vi "Geometry prep.vi"() -> ()   [LabVIEW 2015]
uses:
  <vilib>/Analysis/NI_AALPro.lvlib
panel:
  out "Area vectors, flap (sorted)":sgl[][](array[numeric])=[[-0.030221105, 0.0050799865, 0.0], [-0.025013696, 0.010133014, 0.0], [-0.016425999, 0.015131993, 0.0], [-0.004751401, 0.020000994, 0.0], [0.0092555005, 0.009600005, -0.0], [0.011616802, -0.009600005, 0.0], [0.017089, -0.020627992, 0.0], [0.038450897, -0.029717995, 0.0]]
  out "Area vectors, wing (sorted)":sgl[][](array[numeric])=[[-0.0203481, 0.080010995, 0.0], [-0.0011855003, 0.03999, 0.0], [0.0039664, 0.039116003, -0.0], [0.0067474004, 0.030846998, -0.0], [0.007422101, 0.019963002, -0.0], [0.005573, 0.009961, -0.0], [0.0017389987, 0.0023479997, -0.0], [0.0026417004, 0.0030260002, -0.0], [0.0037459005, 0.003527, -0.0], [0.0068250997, 0.002781997, -0.0], [0.0076412004, -0.0055579967, 0.0], [0.0006181995, -0.0030020003, 0.0], [-1.3899662e-05, -0.0030160001, 0.0], [-0.0003820001, -0.0030109999, 0.0], [-0.0011917998, -0.006011999, 0.0], [-0.0017578002, -0.0068530007, 0.0], [-0.0058059003, -0.022149, 0.0], [-0.0077515002, -0.039984, 0.0], [-0.0046135993, -0.039992005, 0.0], [-0.0017817, -0.03999, 0.0], [0.0030151003, -0.03999099, 0.0], [-0.0051033013, -0.022013, 0.0]]
  in  "Span (m)":dbl=1.0
  in  "Chord (m)":dbl=0.314309
  in  "Clockwise winding?":bool=TRUE
  in  "y/c flap (sorted)":dbl[](array[numeric])=[0.37029770016670227, 0.27414676547050476, 0.194563627243042, 0.1423029601573944, 0.12718598544597626, 0.15663312375545502, 0.19359293580055237, 0.24796299636363983]
  in  "x/c flap (sorted)":dbl[](array[numeric])=[0.9951130747795105, 0.9789506793022156, 0.9467116594314575, 0.8985679745674133, 0.8349331617355347, 0.8043899536132812, 0.8349331617355347, 0.9005628228187561]
  in  "y/c wing (sorted":dbl[](array[numeric])=[-0.055548522621393204, -0.12028767913579941, -0.12405944615602493, -0.1114400178194046, -0.0899726077914238, -0.06635858118534088, -0.04862762242555618, -0.043094854801893234, -0.034690067172050476, -0.022772176191210747, -0.0010575579944998026, 0.0232535507529974, 0.02522040344774723, 0.02517618052661419, 0.023960815742611885, 0.020169006660580635, 0.014576420187950134, -0.0038955300115048885, -0.028557566925883293, -0.04323611408472061, -0.04890473932027817, -0.03931194916367531]
  in  "x/c wing (sorted)":dbl[](array[numeric])=[0.7367812991142273, 0.48221972584724426, 0.3549882471561432, 0.23053745925426483, 0.1323951929807663, 0.06888125836849213, 0.03718951717019081, 0.029719162732362747, 0.020091693848371506, 0.008870252408087254, 1.9099999917671084e-05, 0.01770232431590557, 0.02725343592464924, 0.036849088966846466, 0.04642883315682411, 0.06555650383234024, 0.08735989034175873, 0.15782876312732697, 0.2850411534309387, 0.41227900981903076, 0.5395104885101318, 0.666745126247406]
  # "(Data sorted by winding no.)"
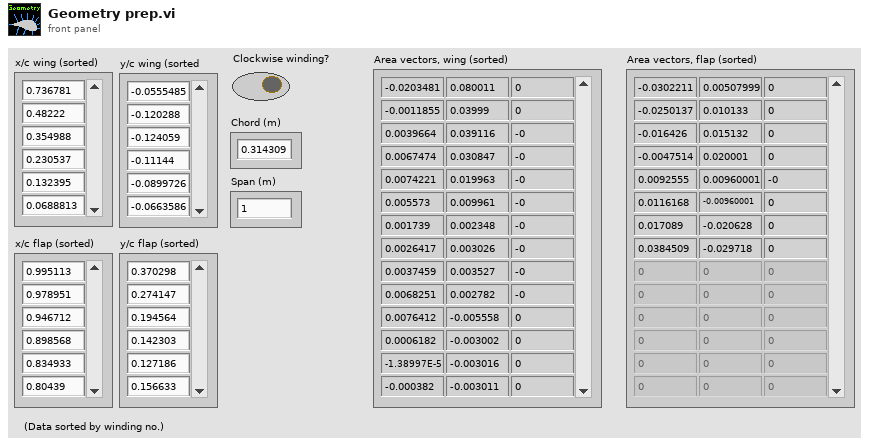
[diagram p1: front panel]
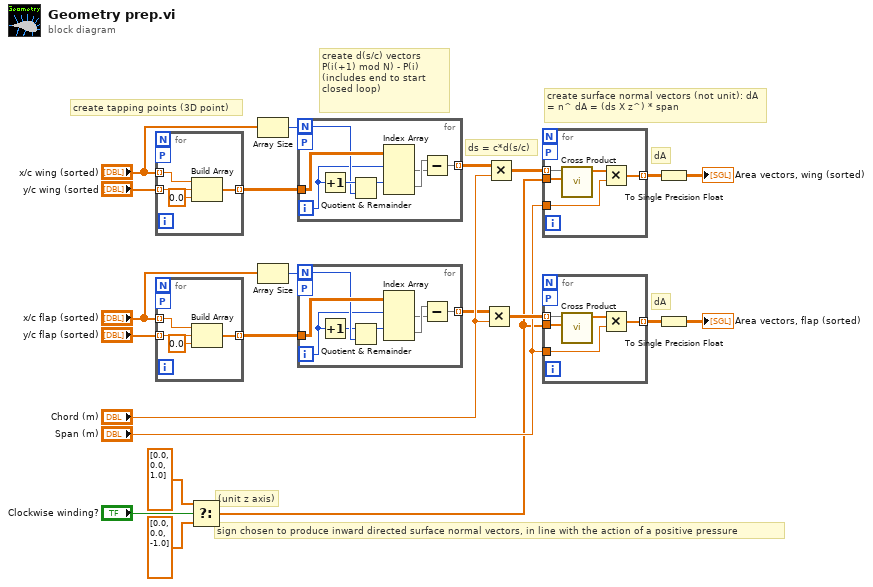
[diagram p0: block diagram]
diagram:
  # "sign chosen to produce inward directed surface normal vectors, in line with the action of a positive pressure"
  # "(unit z axis)"
  # "dA"
  # "dA"
  # "create surface normal vectors (not unit): dA = n^ dA = (ds X z^) * span"
  # "ds = c*d(s/c)"
  # "create d(s/c) vectors P(i(+1) mod N) - P(i)\n(includes end to start closed loop)"
  # "create tapping points (3D point)"
  n1 = for {
    workers-P: _ -> [_]
    tunnel: "x/c wing (sorted)" -> [w26] mode=indexing
    tunnel: "y/c wing (sorted" -> [w25] mode=indexing
    tunnel: [w23] -> w16 mode=indexing
    n2 = Build Array(w26, w25, 0.0 ("element")) -> (w23:dbl[])
  }
  n3 = for {
    workers-P: _ -> [_]
    tunnel: "x/c flap (sorted)" -> [w30] mode=indexing
    tunnel: "y/c flap (sorted)" -> [w29] mode=indexing
    tunnel: [w27] -> w11 mode=indexing
    n4 = Build Array(w30, w29, 0.0 ("element")) -> (w27:dbl[])
  }
  n5 = Select(t=dbl[] [0.0, 0.0, 1.0], s="Clockwise winding?", f=dbl[] [0.0, 0.0, -1.0]) -> (s? t:f=w3:dbl[])
  n6 = Array Size(array="x/c wing (sorted)") -> (size(s)=w2:i32)
  n7 = Array Size(array="x/c flap (sorted)") -> (size(s)=w1:i32)
  n8 = for {
    N: w2 -> [w32]
    tunnel: w16 -> [w37]
    tunnel: [w38] -> w14 mode=indexing
    workers-P: _ -> [_]
    i -> [w31]
    n9 = Increment(x=w31) -> (x+1=w33:i32)
    n10 = Quotient & Remainder(x=w33, y=w32) -> (x-y*floor(x/y)=w34:i32)  [unwired: 1 out]
    n11 = Index Array(array=w37, index (row) #1=w31, index (row) #2=w34) -> (element #1=w35:dbl[], element #2=w36:dbl[])  [unwired: 2 in]
    n12 = Subtract(x=w36, y=w35) -> (x-y=w38:dbl[])
  }
  n13 = for {
    N: w1 -> [w42]
    tunnel: w11 -> [w45]
    tunnel: [w46] -> w10 mode=indexing
    workers-P: _ -> [_]
    i -> [w40]
    n14 = Increment(x=w40) -> (x+1=w41:i32)
    n15 = Quotient & Remainder(x=w41, y=w42) -> (x-y*floor(x/y)=w39:i32)  [unwired: 1 out]
    n16 = Index Array(array=w45, index (row) #1=w40, index (row) #2=w39) -> (element #1=w43:dbl[], element #2=w44:dbl[])  [unwired: 2 in]
    n17 = Subtract(x=w44, y=w43) -> (x-y=w46:dbl[])
  }
  n18 = Multiply(x=w10, y="Chord (m)") -> (x*y=w12:dbl[][])
  n19 = Multiply(x=w14, y="Chord (m)") -> (x*y=w9:dbl[][])
  n20 = for {
    tunnel: w9 -> [w51] mode=indexing
    tunnel: w3 -> [w50]
    workers-P: _ -> [_]
    tunnel: "Span (m)" -> [w48]
    tunnel: [w47] -> w7 mode=indexing
    n21 = call <vilib>:"Cross Product.vi"("B Vector"=w50, "A Vector"=w51) -> ("Cross Product"=w49:dbl[])  [unwired: 8 in, 1 out]
    n22 = Multiply(x=w49, y=w48) -> (x*y=w47:dbl[])
  }
  n23 = for {
    tunnel: w12 -> [w56] mode=indexing
    tunnel: w3 -> [w55]
    workers-P: _ -> [_]
    tunnel: "Span (m)" -> [w53]
    tunnel: [w52] -> w6 mode=indexing
    n24 = call <vilib>:"Cross Product.vi"("B Vector"=w55, "A Vector"=w56) -> ("Cross Product"=w54:dbl[])  [unwired: 8 in, 1 out]
    n25 = Multiply(x=w54, y=w53) -> (x*y=w52:dbl[])
  }
  n26 = To Single Precision Float(number=w7) -> (single precision float=→"Area vectors, wing (sorted)":sgl[][])
  n27 = To Single Precision Float(number=w6) -> (single precision float=→"Area vectors, flap (sorted)":sgl[][])
